vi "Check Count.vi"(5 "source vi name":string, 6 "count power of 2":i16, 8 "error in (no error)":errorcluster, 9 "offset (0)":u64 format="%d bytes", 10 "count (-1: rest)":i64=-1 format="%d elements", 11 "Pointer in":refnum<class "Pointer.lvclass">) -> (0 "error out":errorcluster, 1 "offset":u64 format="%d bytes", 2 "count":u64 format="%d elements", 3 "Pointer out":refnum<class "Pointer.lvclass">)   [LabVIEW 2017, in "Memory Manager.lvlib" / "Pointer.lvclass"]
uses:
  Pointer.lvclass
  Out of Bounds.vi
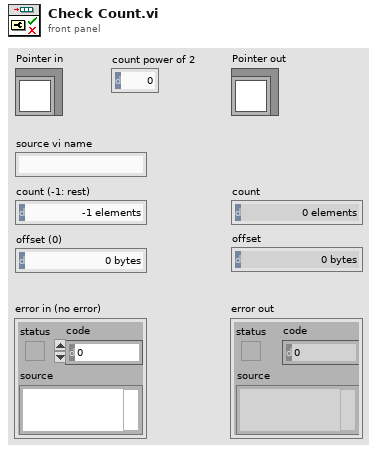
[diagram p1: front panel]
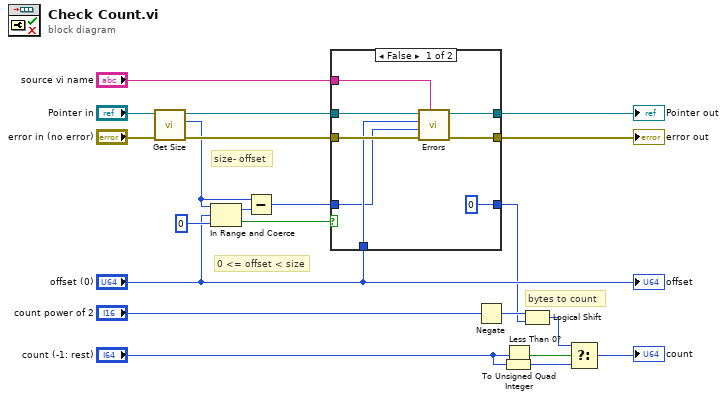
[diagram p0: block diagram]
diagram:
  # "bytes to count"
  # "size- offset"
  # "0 <= offset < size"
  n1 = call "Get Size.vi"("Pointer in"="Pointer in") -> ("size"=w6:u64, "Pointer out"=w13:refnum<class "Pointer.lvclass">)  [unwired: 9 in]
  n2 = In Range and Coerce(upper limit=w6, x="offset (0)", lower limit=u64 0) -> (coerced(x)=w5:u64, In Range?=w14:bool)
  n3 = Subtract(x=w6, y=w5) -> (x-y=w4:u64)
  n4 = case shown="False" w14 {
    tunnel: w13 -> [w28 w31]
    tunnel: "error in (no error)" -> [w27 w30]
    tunnel: [w26 w31] -> w11
    tunnel: [w25 w30] -> w10
    tunnel: "source vi name" -> [w24 _]
    tunnel: "offset (0)" -> [w23 _]
    tunnel: w4 -> [w22 w29]
    tunnel: [u64 0 ("t") w29] -> w1
    frame False {
      n5 = call-poly "Errors.vi"("error source vi name"=w24, "error in (no error)"=w27, "size"=w22, "offset"=w23, "Pointer in"=w28) -> ("error out"=w25:errorcluster, "Pointer out"=w26:refnum<class "Pointer.lvclass">)  [unwired: 5 in]
    }
    frame True {
    }
  }
  "error out" <- w10
  "Pointer out" <- w11
  n6 = Negate(x="count power of 2") -> (-x=w8:i16)
  n7 = To Unsigned Quad Integer(1:"count (-1: rest)") -> (0:w18:u64)
  n8 = Less Than 0?(x="count (-1: rest)") -> (x < 0?=w16:bool)
  n9 = Logical Shift(y=w8, x=w1) -> (x << y=w3:u64)
  n10 = Select(t=w3, s=w16, f=w18) -> (s? t:f=→"count":u64)
  "offset" <- "offset (0)"
